vi "Concatenate.vi"() -> ()   [LabVIEW 2021]
panel:
  out "Array":i32[](array[numeric])
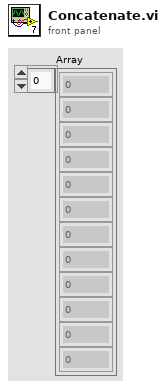
[diagram p1: front panel]
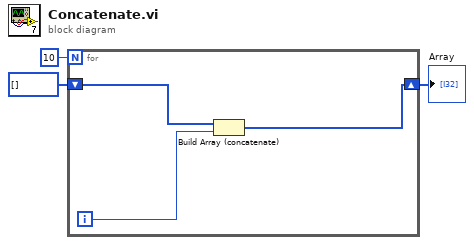
[diagram p0: block diagram]
diagram:
  n1 = for {
    N: 10 -> [_]
    shift-right: [w4] -> w1
    shift-left: i32[] [] -> [w6]
    i -> [w5]
    n2 = Build Array (concatenate)(w6, w5) -> (w4:i32[])
  }
  "Array" <- w1
